vi "ReadSocket.vi"(8 "error in (no error)":errorcluster, 11 "reference in":refnum<class "WebSocket.lvclass">) -> (0 "error out":errorcluster, 2 "Socket":refnum<k5>, 3 "reference out":refnum<class "WebSocket.lvclass">)   [LabVIEW 2017, in "WebSocket.lvclass"]
uses:
  WebSocket.lvclass
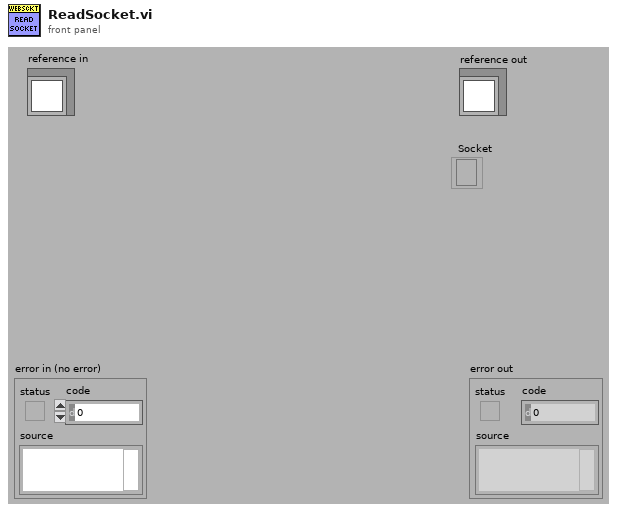
[diagram p1: front panel]
types:
  T1 = typedef "WebSocket.lvclass/ObjectAttributes.ctl" = cluster{"Socket":refnum<k5>, "Thread":refnum<vi>, "From Socket":refnum<queue>, "To Socket":refnum<queue>, "Rx Stats in Progress":variant, "Rx Stats":variant, "Tx Stats in Progress":variant, "Tx Stats":variant}
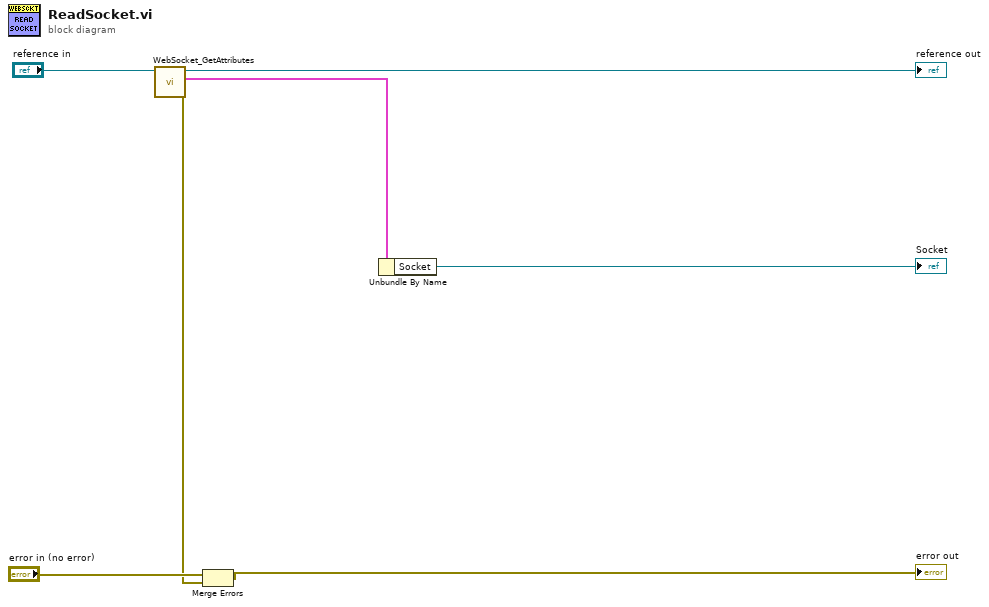
[diagram p0: block diagram]
diagram:
  n1 = call "WebSocket_GetAttributes.vi"("reference in"="reference in") -> ("error out"=w2:errorcluster, "Data"=w4:T1, "reference out"=→"reference out":refnum<class "WebSocket.lvclass">)  [unwired: 7 in, 1 out]
  n2 = Merge Errors("error in (no error)", w2) -> (→"error out":errorcluster)
  n3 = Unbundle By Name(w4) -> ("Socket"=→"Socket":refnum<k5>)
